vi "posRaw_to_useful.vi"(8 "wheelDiameter (in)":dbl, 10 "ticksPerRot":dbl=4096.0, 11 "rawInput":dbl) -> (0 "feet":dbl, 3 "rotations":dbl)   [LabVIEW 2017]
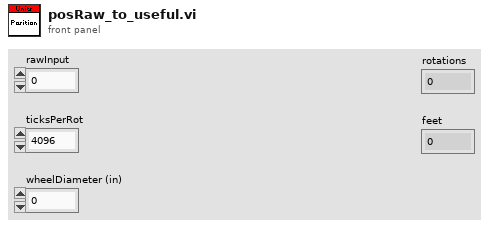
[diagram p1: front panel]
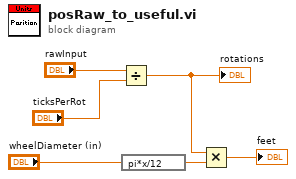
[diagram p0: block diagram]
diagram:
  n1 = Divide(x="rawInput", y="ticksPerRot") -> (x/y=w2:dbl)
  "rotations" <- w2
  n2 = expression code="pi*x/12"("wheelDiameter (in)") -> (w1:dbl)
  n3 = Multiply(x=w2, y=w1) -> (x*y=→"feet":dbl)
